vi "GetTrigTmstmp.vi"(8 "error in (no error)":errorcluster, 10 "TriggerName":T1={"TriggerName"="", "Timeout (s)"=1.0}, 11 "PXI_MultiTrig in":refnum<class "PXI_MultiTrig.lvclass">) -> (0 "error out":errorcluster, 2 "Timestamp":dbl format="%_6f", 3 "PXI_MultiTrig out":refnum<class "PXI_MultiTrig.lvclass">)   [LabVIEW 2014, in "SyncPlugins.lvlib" / "PXI_MultiTrig.lvclass"]
uses:
  PXI_MultiTrig.lvclass
  SyncPluginBase/Typedefs/clGetTrigTmstmp.ctl
  PXI_MultiTrig.lvclass/PXI_MultiTrig.ctl
  SyncPluginBase/SyncPluginBase.lvclass/SyncPluginBase.ctl
  SyncPluginBase/Accessors/Read PPSTime.vi
  Accessors/Read RefClkSession.vi
  Accessors/Read Triggers.vi
  <vilib>/Utility/error.llb/Error Cluster From Error Code.vi
  <instrlib>/niSync/niSync.llb/niSync Read Trigger Time Stamp (Single).vi
  <vilib>/ErrorRing/Error Ring.xnode
  SyncPluginBase/SyncPluginBase.lvclass
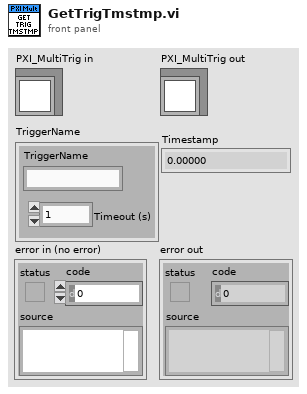
[diagram p1: front panel]
types:
  T1 = typedef "SyncPlugins.lvlib/SyncPluginBase.lvclass/clGetTrigTmstmp.ctl" = cluster{"TriggerName":string, "Timeout (s)":dbl}
  T2 = typedef "SyncPlugins.lvlib/PXI_MultiTrig.lvclass/clTrigger.ctl" = cluster{"Name":string, "DestTerm":string, "SrcTerm":string, "SyncClk":string, "Edge":i32, "Invert?":i32, "Initiated":bool, "Type":string, "TrigTime":bool}
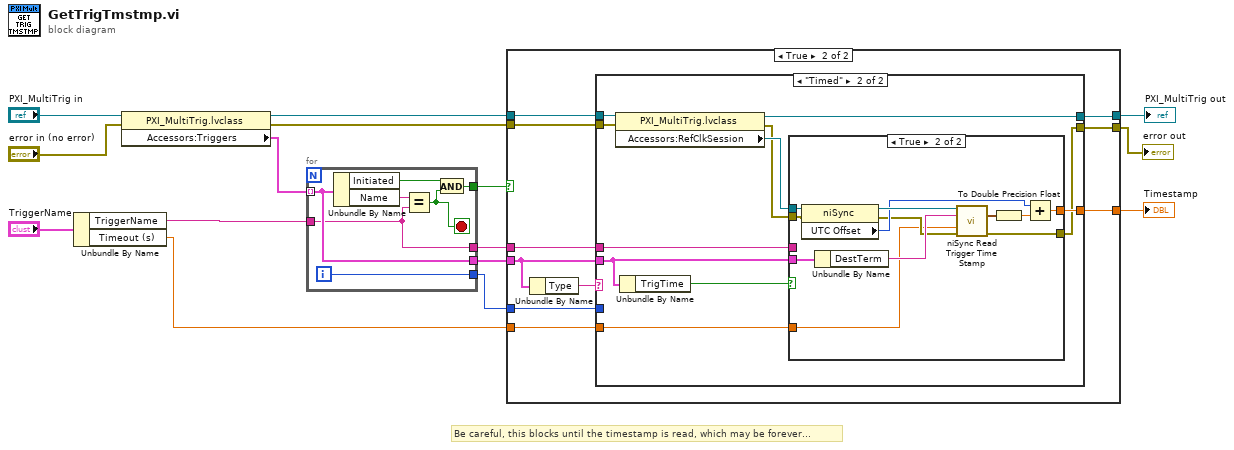
[diagram p0: block diagram]
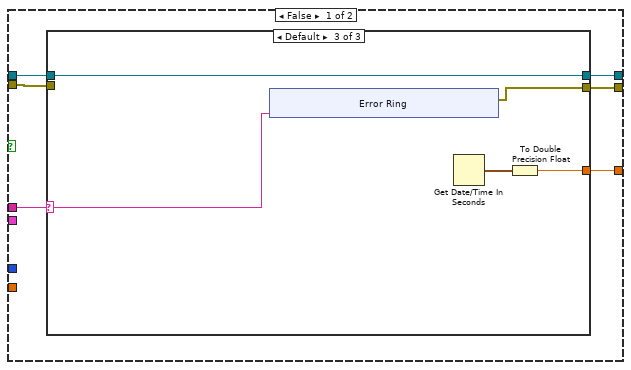
[diagram p2: hidden frame]
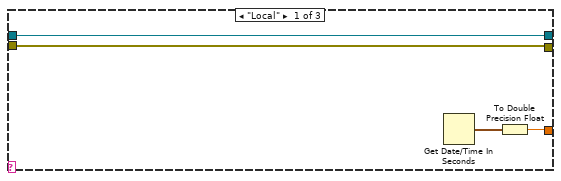
[diagram p3: hidden frame]
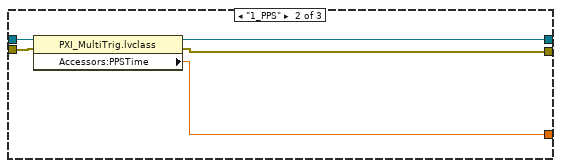
[diagram p4: hidden frame]
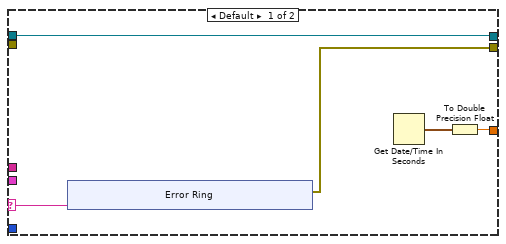
[diagram p5: hidden frame]
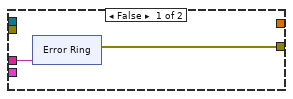
[diagram p6: hidden frame]
diagram:
  # "Be careful, this blocks until the timestamp is read, which may be forever..."
  n1 = Unbundle By Name("TriggerName") -> ("TriggerName"=w2:string, "Timeout (s)"=w1:dbl)
  n2 = property class="PXI_MultiTrig.lvclass"(reference="PXI_MultiTrig in", error in="error in (no error)") -> (reference out=w10:refnum<class "PXI_MultiTrig.lvclass">, error out=w6:errorcluster, "Accessors:Triggers"=w12:T2[])
  n3 = for {
    tunnel: w12 -> [w21] mode=indexing
    tunnel: [w21] -> w8
    tunnel: [w18] -> w11
    tunnel: [w17] -> w7
    tunnel: w2 -> [w16]
    tunnel: [w16] -> w9
    i -> [w17]
    stop <- w20 stop-if-true
    n4 = Unbundle By Name(w21) -> ("Initiated"=w19:bool, "Name"=w22:string)
    n5 = Equal?(x=w22, y=w16) -> (x = y?=w20:bool)
    n6 = And(x=w19, y=w20) -> (x .and. y?=w18:bool)
  }
  n7 = case shown="True" w11 {
    tunnel: w10 -> [w26 w54]
    tunnel: w9 -> [w28 w57]
    tunnel: [w25 w51] -> w4
    tunnel: [w27 w58] -> w3
    tunnel: w8 -> [_ w55]
    tunnel: w7 -> [_ w56]
    tunnel: w6 -> [w24 w53]
    tunnel: [w23 w52] -> w5
    tunnel: w1 -> [_ w50]
    frame False {
      n8 = case shown="Default" w28 {
        selector: w28 -> [_ _ w42]
        tunnel: [w29 w35 w41] -> w27
        tunnel: w26 -> [w30 w37 w40]
        tunnel: [w30 w34 w40] -> w25
        tunnel: w24 -> [w29 w36 _]
        tunnel: [w31 w33 w38] -> w23
        frame "Local" {
          n9 = Get Date/Time In Seconds() -> (seconds since 1Jan1904=w32:timestamp)
          n10 = To Double Precision Float(number=w32) -> (double precision float=w31:dbl)
        }
        frame "1_PPS" {
          n11 = property class="PXI_MultiTrig.lvclass"(reference=w37, error in=w36) -> (reference out=w34:refnum<class "PXI_MultiTrig.lvclass">, error out=w35:errorcluster, "Accessors:PPSTime"=w33:dbl)
        }
        frame Default {
          n12 = xnode "Error Ring"("parameter 0"=w42) -> ("error out"=w41:errorcluster)
          n13 = Get Date/Time In Seconds() -> (seconds since 1Jan1904=w39:timestamp)
          n14 = To Double Precision Float(number=w39) -> (double precision float=w38:dbl)
        }
      }
    }
    frame True {
      n15 = Unbundle By Name(w55) -> ("Type"=w59:string)
      n16 = case shown="\"Timed\"" w59 {
        selector: w59 -> [w64 _]
        tunnel: [w63 w73] -> w58
        tunnel: w57 -> [_ w78]
        tunnel: w56 -> [_ _]
        tunnel: w55 -> [_ w77]
        tunnel: w54 -> [w62 w82]
        tunnel: w53 -> [_ w81]
        tunnel: [w60 w75] -> w52
        tunnel: [w62 w74] -> w51
        tunnel: w50 -> [_ w72]
        frame Default {
          n17 = xnode "Error Ring"("parameter 0"=w64) -> ("error out"=w63:errorcluster)
          n18 = Get Date/Time In Seconds() -> (seconds since 1Jan1904=w61:timestamp)
          n19 = To Double Precision Float(number=w61) -> (double precision float=w60:dbl)
        }
        frame "Timed" {
          n20 = property class="PXI_MultiTrig.lvclass"(reference=w82, error in=w81) -> (reference out=w74:refnum<class "PXI_MultiTrig.lvclass">, error out=w76:errorcluster, "Accessors:RefClkSession"=w79:refnum<k15>)
          n21 = Unbundle By Name(w77) -> ("TrigTime"=w80:bool)
          n22 = case shown="True" w80 {
            tunnel: w79 -> [_ w102]
            tunnel: w78 -> [w84 _]
            tunnel: w77 -> [_ w103]
            tunnel: w76 -> [_ w99]
            tunnel: [_ w95] -> w75
            tunnel: [w83 w93] -> w73
            tunnel: w72 -> [_ w92]
            frame False {
              n23 = xnode "Error Ring"("parameter 0"=w84) -> ("error out"=w83:errorcluster)
            }
            frame True {
              n24 = property class="niSync"(reference=w102, error in=w99) -> (reference out=w100:refnum<k15>, error out=w94:errorcluster, "UTC Offset"=w96:i32)
              n25 = Unbundle By Name(w103) -> ("DestTerm"=w101:string)
              n26 = call-poly <instrlib>:"niSync Read Trigger Time Stamp.vi"("instrument handle"=w100, "terminal"=w101, "timeout"=w92, "error in (no error)"=w94) -> ("time stamp out"=w98:timestamp, "error out"=w93:errorcluster)  [unwired: 8 in, 2 out]
              n27 = To Double Precision Float(number=w98) -> (double precision float=w97:dbl)
              n28 = Add(x=w96, y=w97) -> (x+y=w95:dbl)
            }
          }
        }
      }
    }
  }
  "error out" <- w3
  "PXI_MultiTrig out" <- w4
  "Timestamp" <- w5
